vi "decodeUInt.vi"(8 "error in (no error)":errorcluster, 10 "ByteArray":u8[](array[numeric]) format="%.0x") -> (0 "error out":errorcluster, 1 "uint":u64, 2 "variant":variant, 3 "RemainingBytes":u8[](array[numeric]), 5 "Type":string)   [LabVIEW 2016, in "MsgPack.lvlib"]
uses:
  MsgPack.lvlib
  <vilib>/Utility/error.llb/Error Cluster From Error Code.vi
  <vilib>/ErrorRing/Error Ring.xnode
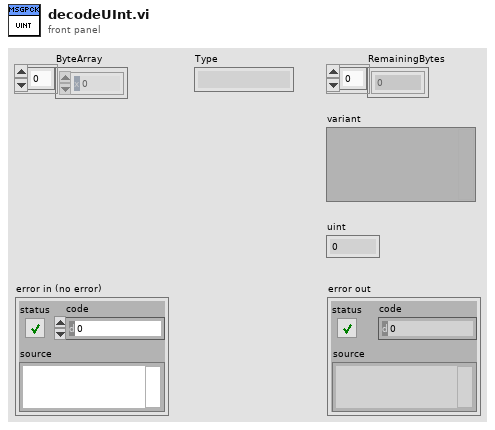
[diagram p1: front panel]
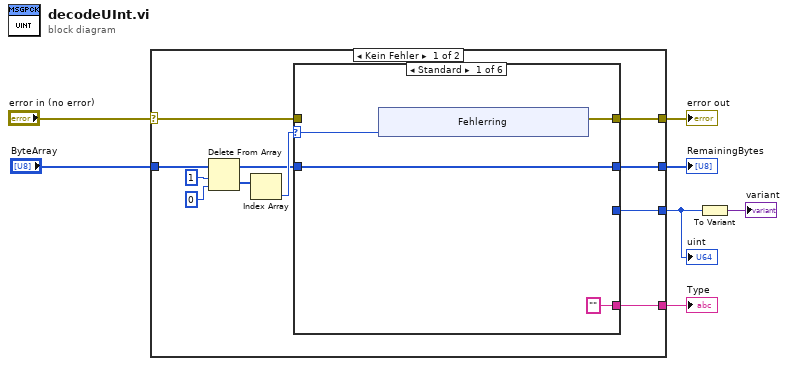
[diagram p0: block diagram]
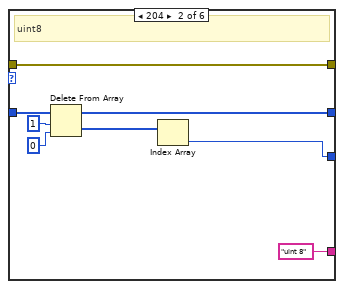
[diagram p2: hidden frame]
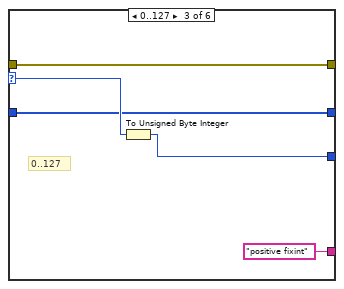
[diagram p3: hidden frame]
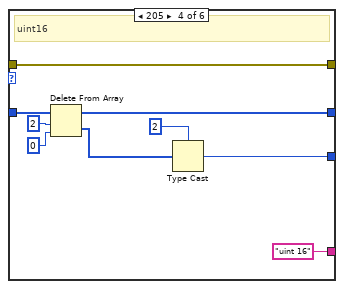
[diagram p4: hidden frame]
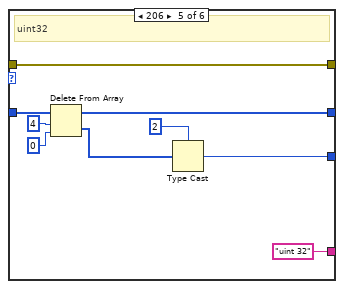
[diagram p5: hidden frame]
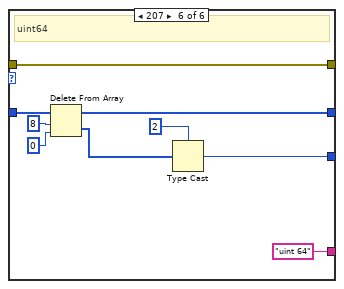
[diagram p6: hidden frame]
diagram:
  n1 = case shown="Kein Fehler" "error in (no error)" {
    selector: "error in (no error)" -> [w8 w71]
    tunnel: [w18 w71] -> w6
    tunnel: [w16 _] -> w5
    tunnel: [w15 _] -> w4
    tunnel: "ByteArray" -> [w12 w70]
    tunnel: [w10 w70] -> w2
    frame No Error {
      n2 = Delete From Array(array=w12, length=1, index=0) -> (deleted portion=w13:u8[], array with subset deleted=w11:u8[])
      n3 = Index Array(array=w13) -> (element=w17:u8)  [unwired: 1 in]
      n4 = case shown="Standard" w17 {
        selector: w17 -> [w20 _ w42 _ _ _]
        tunnel: [w21 w37 w38 w51 w60 w69] -> w18
        tunnel: w8 -> [_ w37 w38 w51 w60 w69]
        tunnel: ["" "uint 8" "positive fixint" "uint 16" "uint 32" "uint 64"] -> w16
        tunnel: [_ w35 w41 w49 w58 w67] -> w15
        tunnel: w11 -> [w19 w34 w40 w47 w55 w65]
        tunnel: [w19 w31 w40 w44 w53 w62] -> w10
        frame Default {
          n5 = xnode "Fehlerring"("Parameter 0"=w20) -> ("Fehler (Ausgang)"=w21:errorcluster)
        }
        frame 204 {
          # "uint8"
          n6 = Delete From Array(array=w34, length=1, index=0) -> (deleted portion=w32:u8[], array with subset deleted=w31:u8[])
          n7 = Index Array(array=w32) -> (element=w35:u8)  [unwired: 1 in]
        }
        frame 0..127 {
          # "0..127"
          n8 = To Unsigned Byte Integer(number=w42) -> (unsigned 8bit integer=w41:u8)
        }
        frame 205 {
          # "uint16"
          n9 = Delete From Array(array=w47, length=2, index=0) -> (deleted portion=w45:u8[], array with subset deleted=w44:u8[])
          n10 = Type Cast(type=u16 2 ("length"), x=w45) -> (*(type *) &x=w49:u16)
        }
        frame 206 {
          # "uint32"
          n11 = Delete From Array(array=w55, length=4, index=0) -> (deleted portion=w54:u8[], array with subset deleted=w53:u8[])
          n12 = Type Cast(type=u32 2 ("length"), x=w54) -> (*(type *) &x=w58:u32)
        }
        frame 207 {
          # "uint64"
          n13 = Delete From Array(array=w65, length=8, index=0) -> (deleted portion=w63:u8[], array with subset deleted=w62:u8[])
          n14 = Type Cast(type=u64 2 ("length"), x=w63) -> (*(type *) &x=w67:u64)
        }
      }
    }
    frame Error {
    }
  }
  "error out" <- w6
  "Type" <- w5
  "uint" <- w4
  "RemainingBytes" <- w2
  n15 = To Variant(anything=w4) -> (Variant=→"variant":variant)
